vi "myRIO_BRig_RT_dataCurrent_Tcycle_cue.vi"() -> (2 "output_Tcycle_cue":i32)   [LabVIEW 2014]
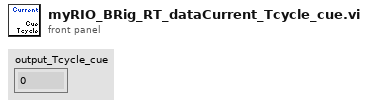
[diagram p1: front panel]
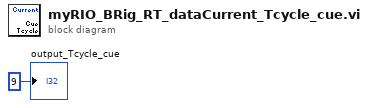
[diagram p0: block diagram]
diagram:
  "output_Tcycle_cue" <- 9 ("output_iBlock")
